vi "Ej 15 DAQ.vi"() -> ()   [LabVIEW 2021]
panel:
  out "XY Graph 2":cluster{dbl[], dbl[]}[](graph)
  in  "stop":bool
  out "Array 2":dbl[](array[numeric])
  out "Array":dbl[](array[numeric])
  out "Waveform Chart":dynamicdata(graph)
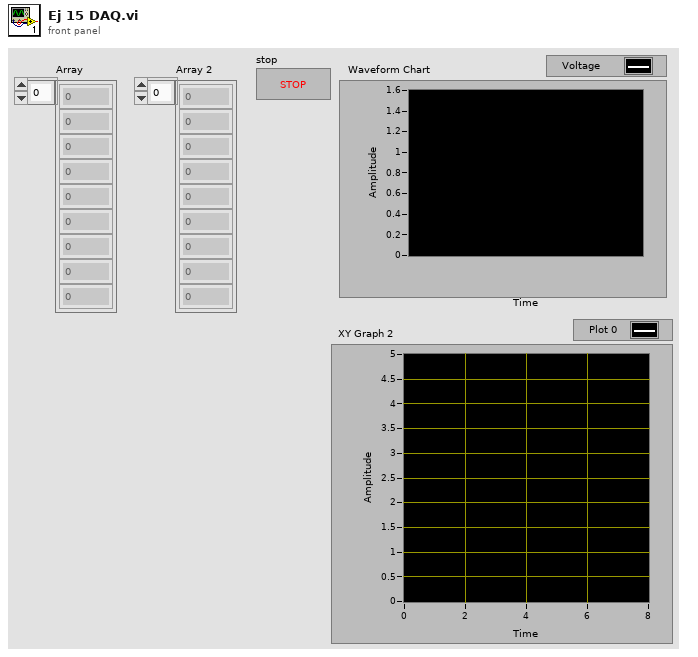
[diagram p1: front panel]
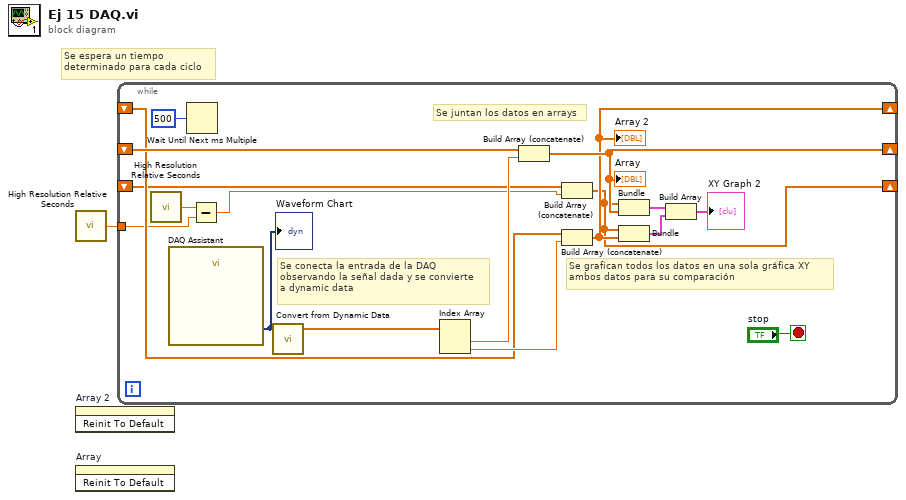
[diagram p0: block diagram]
diagram:
  # "Se espera un tiempo\ndeterminado para cada ciclo"
  n1 = call <vilib>:"High Resolution Relative Seconds.vi"() -> ("relative seconds"=w1:dbl)
  n2 = invoke on="Array 2" class="Arr (strict)" method="Reinit To Default"() -> ()  [unwired: 3 in, 3 out]
  n3 = invoke on="Array" class="Arr (strict)" method="Reinit To Default"() -> ()  [unwired: 3 in, 3 out]
  n4 = while {
    shift-right: [w8] -> _
    shift-left: _ -> [w16]
    shift-right: [w7] -> _
    shift-left: _ -> [w15]
    tunnel: w1 -> [w10]
    shift-right: [w6] -> _
    shift-left: _ -> [w9]
    stop <- "stop" stop-if-true
    # "Se grafican todos los datos en una sola gráfica XY \nambos datos para su comparación"
    # "Se juntan los datos en arrays"
    # "Se conecta la entrada de la DAQ\nobservando la señal dada y se convierte\na dynamic data"
    n5 = call <vilib>:"High Resolution Relative Seconds.vi"() -> ("relative seconds"=w11:dbl)
    n6 = call "DAQ Assistant"() -> ("data"=w13:dynamicdata)  [unwired: 17 in, 2 out]
    "Waveform Chart" <- w13
    n7 = Wait Until Next ms Multiple(millisecond multiple=u32 500) -> ()  [unwired: 1 out]
    n8 = Subtract(x=w11, y=w10) -> (x-y=w12:dbl)
    n9 = call "Convert from Dynamic Data"("Dynamic Data Type"=w13) -> ("Array"=w19:dbl[])  [unwired: 3 in]
    n10 = Index Array "Index Array"(array=w19) -> (element #1=w18:dbl, element #2=w17:dbl)  [unwired: 2 in]
    n11 = Build Array (concatenate) "Build Array"(w16, w18) -> (w8:dbl[])
    "Array" <- w8
    n12 = Build Array (concatenate)(w9, w12) -> (w6:dbl[])
    n13 = Build Array (concatenate)(w15, w17) -> (w7:dbl[])
    "Array 2" <- w7
    n14 = Bundle(w6, w8) -> (w4:cluster{dbl[], dbl[]})  [unwired: 1 in]
    n15 = Bundle(w6, w7) -> (w5:cluster{dbl[], dbl[]})  [unwired: 1 in]
    n16 = Build Array(w4, w5) -> (→"XY Graph 2":cluster{dbl[], dbl[]}[])
  }
